vi "templates add INI as new.vi"(6 "import?":bool, 7 "name":string, 8 "error in":errorcluster, 9 "user":string, 10 "INI File Content":string, 11 "Connection Refnum":T1) -> (0 "error out":errorcluster, 1 "Parameters":T3, 2 "updated Template Record":T2, 3 "Connection Refnum 2":T1, 4 "Layout Filess":string[](array[string]))   [LabVIEW 2011]
uses:
  Addons/internet/utils/keyedarr.llb/Keyed Array.ctl
  server/database/Templates/Template Record.ctl
  SI.LIB/ODBC/SQL Controls/Connection Refnum.ctl
panel:
  out "Temp Folder":path
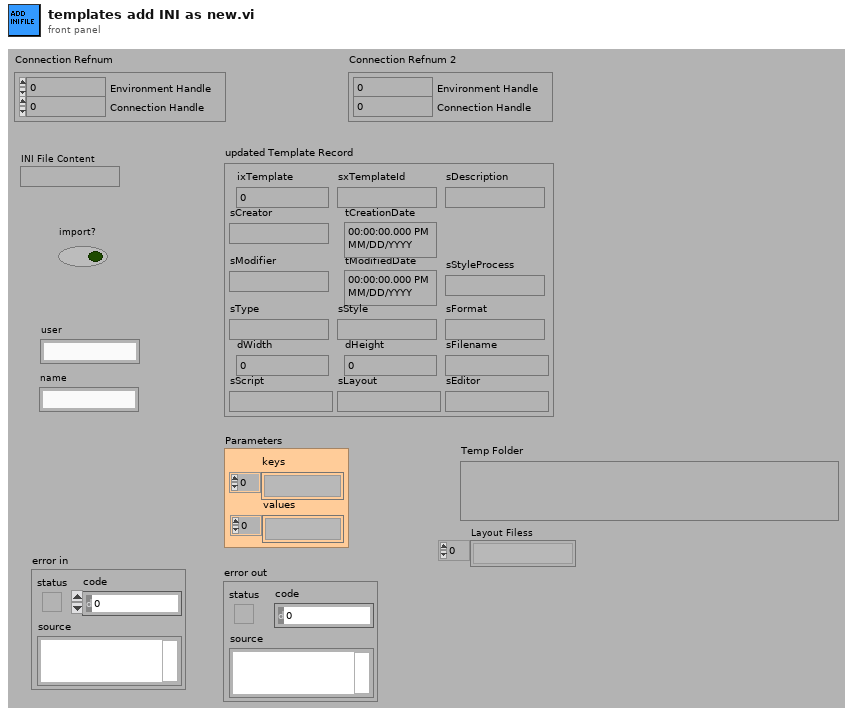
[diagram p1: front panel]
types:
  T1 = typedef "Connection Refnum.ctl" = cluster{"Environment Handle":i32, "Connection Handle":i32}
  T2 = typedef "Template Record.ctl" = cluster{"ixTemplate":i32, "sxTemplateId":string, "sDescription":string, "sCreator":string, "tCreationDate":timestamp, "sModifier":string, "tModifiedDate":timestamp, "sType":string, "sStyle":string, "sFormat":string, "dWidth":dbl, "dHeight":dbl, "sFilename":string, "sScript":string, "sLayout":string, "sEditor":string, "sStyleProcess":string}
  T3 = typedef "Keyed Array.ctl" = cluster{"keys":string[], "values":string[]}
  T4 = enum16{"open", "replace", "create", "open or create", "replace or create", "replace or create with confirmation"}
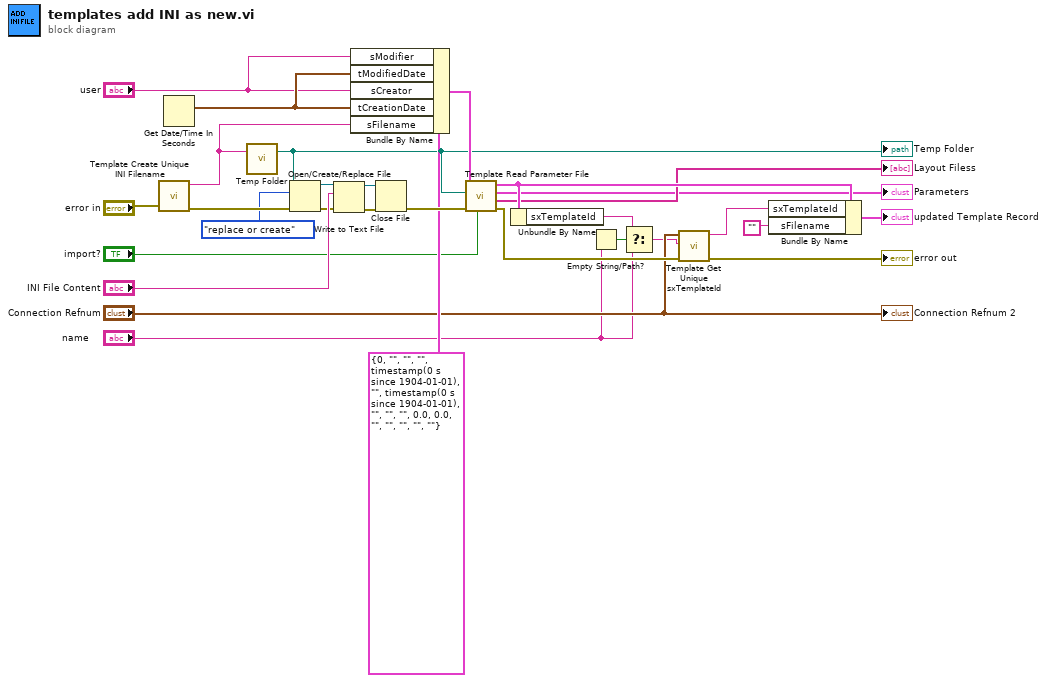
[diagram p0: block diagram]
diagram:
  n1 = call "Template Create Unique INI Filename.vi"("error in (no error)"="error in") -> ("error out"=w29:errorcluster, "INI Name"=w3:string)  [unwired: 9 out]
  n2 = Get Date/Time In Seconds() -> (seconds since 1Jan1904=w7:timestamp)
  n3 = call "Temp Folder.vi"("Relative Path (\"\")"=w3) -> ("Temp Folder"=w14:path)  [unwired: 2 in]
  "Temp Folder" <- w14
  n4 = Open/Create/Replace File(file path (use dialog)=w14, error in=w29, operation (0:open)=T4."replace or create") -> (refnum out=w21:refnum<file>, error out=w22:errorcluster)  [unwired: 4 out]
  n5 = Write to Text File(file (use dialog)=w21, text="INI File Content", error in=w22) -> (refnum out=w23:refnum<file>, error out=w24:errorcluster)  [unwired: 2 out]
  n6 = Bundle By Name(cluster=T2 {"ixTemplate"=0, "sxTemplateId"="", "sDescription"="", "sCreator"="", "tCreationDate"=timestamp(0 s since 1904-01-01), "sModifier"="", "tModifiedDate"=timestamp(0 s since 1904-01-01), "sType"="", "sStyle"="", "sFormat"="", "dWidth"=0.0, "dHeight"=0.0, "sFilename"="", "sScript"="", "sLayout"="", "sEditor"="", "sStyleProcess"=""} ("Template Record"), "sModifier"="user", "tModifiedDate"=w7, "sCreator"="user", "tCreationDate"=w7, "sFilename"=w3) -> (w26:T2)
  n7 = Close File(refnum=w23, error in=w24) -> (error out=w27:errorcluster)  [unwired: 1 out]
  n8 = call "Template Read Parameter File.vi"("Import?"="import?", "error in (no error)"=w27, "Alternate Path (\"\")"=w14, "Template Record"=w26) -> ("error out"=w18:errorcluster, "Layout Files"=→"Layout Filess":string[], "Parameters"=→"Parameters":T3, "updated Template Record"=w17:T2)  [unwired: 4 out]
  n9 = Unbundle By Name(w17) -> ("sxTemplateId"=w11:string)
  n10 = Empty String/Path?(string/path="name") -> (empty?=w10:bool)
  n11 = Select(t=w11, s=w10, f="name") -> (s? t:f=w9:string)
  n12 = call "Template Get Unique sxTemplateId.vi"("error in"=w18, "sxTemplateId proposed"=w9, "Connection Refnum"="Connection Refnum") -> ("error out"=→"error out":errorcluster, "sxTemplateId"=w16:string)  [unwired: 7 out]
  n13 = Bundle By Name(cluster=w17, "sxTemplateId"=w16, "sFilename"="") -> (→"updated Template Record":T2)
  "Connection Refnum 2" <- "Connection Refnum"
